vi "Data set defs.vi"(8 "error in (no error)":errorcluster, 11 "MB_TCP in":refnum<class "MB_TCP.lvclass">) -> (0 "error out":errorcluster, 3 "MB_TCP out":refnum<class "MB_TCP.lvclass">)   [LabVIEW 2019, in "MB_TCP.lvclass"]
uses:
  MB_TCP.lvclass
  MB_TCP.lvclass/MB_TCP.ctl
  ICPCON Registers/ICPCON Registers.lvlib
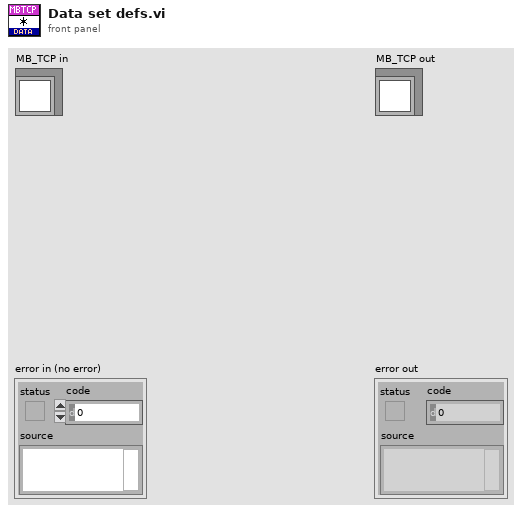
[diagram p1: front panel]
types:
  T1 = typedef "ICPCON Registers.lvlib/ICPCON Data.ctl" = cluster{"UTF":refnum<data-value>, "DI":refnum<data-value>, "DW":refnum<data-value>, "DO":refnum<data-value>, "IR":refnum<data-value>, "WR":refnum<data-value>, "OR":refnum<data-value>, "modified":refnum<data-value>}
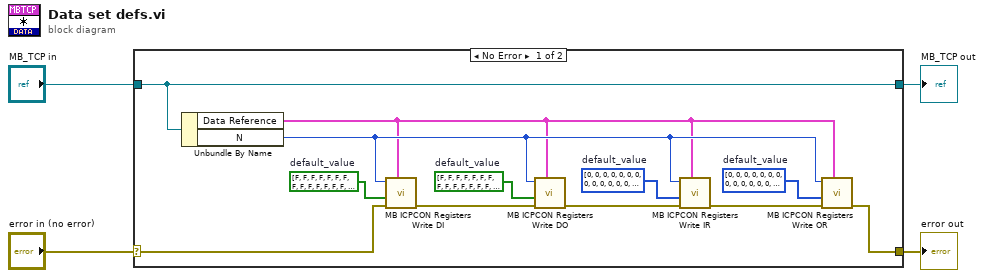
[diagram p0: block diagram]
diagram:
  n1 = case shown="No Error" "error in (no error)" {
    selector: "error in (no error)" -> [w6 w17]
    tunnel: [w5 w17] -> w3
    tunnel: [w16 w18] -> w1
    tunnel: "MB_TCP in" -> [w16 w18]
    frame No Error {
      w12 = u16[] [0, 0, 0, 0, 0, 0, 0, 0, 0, 0, 0, 0, 0, 0, 0, 0, 0, 0, 0, 0]  # default_value
      w13 = bool[] [FALSE, FALSE, FALSE, FALSE, FALSE, FALSE, FALSE, FALSE, FALSE, FALSE, FALSE, FALSE, FALSE, FALSE, FALSE, FALSE, FALSE, FALSE, FALSE, FALSE, FALSE, FALSE, FALSE, FALSE, FALSE, FALSE, FALSE, FALSE, FALSE, FALSE, FALSE, FALSE]  # default_value
      w14 = bool[] [FALSE, FALSE, FALSE, FALSE, FALSE, FALSE, FALSE, FALSE, FALSE, FALSE, FALSE, FALSE, FALSE, FALSE, FALSE, FALSE, FALSE, FALSE, FALSE, FALSE, FALSE, FALSE, FALSE, FALSE, FALSE, FALSE, FALSE, FALSE, FALSE, FALSE, FALSE, FALSE]  # default_value
      w15 = u16[] [0, 0, 0, 0, 0, 0, 0, 0, 0, 0, 0, 0, 0, 0, 0, 0, 0, 0, 0, 0]  # default_value
      n2 = Unbundle By Name(w16) -> ("Data Reference"=w10:T1, "N"=w11:i32)
      n3 = call "MB ICPCON Registers Write DI.vi"("Data Reference"=w10, "error in (no error)"=w6, "Bits In"=w13, "N"=w11) -> ("error out"=w9:errorcluster)  [unwired: 7 in]
      n4 = call "MB ICPCON Registers Write DO.vi"("Data Reference"=w10, "error in (no error)"=w9, "Bits In"=w14, "N"=w11) -> ("error out"=w8:errorcluster)  [unwired: 7 in]
      n5 = call "MB ICPCON Registers Write IR.vi"("Data Reference"=w10, "error in (no error)"=w8, "Words In"=w15, "N"=w11) -> ("error out"=w7:errorcluster)  [unwired: 7 in]
      n6 = call "MB ICPCON Registers Write OR.vi"("Data Reference"=w10, "error in (no error)"=w7, "Words In"=w12, "N"=w11) -> ("error out"=w5:errorcluster)  [unwired: 7 in]
    }
    frame Error {
    }
  }
  "error out" <- w3
  "MB_TCP out" <- w1
